vi "Save Setup.vi"(8 "error in (no error)":errorcluster, 11 "JSON in":refnum<class "JSON.lvclass">) -> (0 "error out":errorcluster, 3 "JSON out":refnum<class "JSON.lvclass">)   [LabVIEW 2018, in "JSON.lvclass"]
uses:
  JSON.lvclass
  JSON.lvclass/JSON.ctl
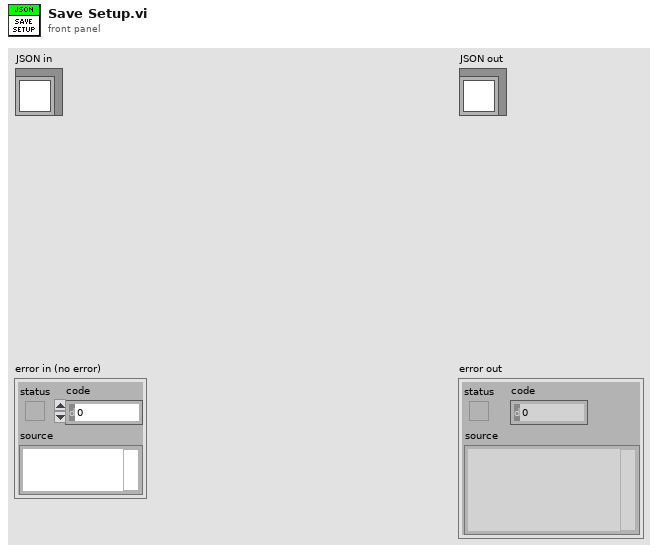
[diagram p1: front panel]
types:
  T1 = enum16{"open", "replace", "create", "open or create", "replace or create", "replace or create with confirmation"}
  T2 = cluster{"Exposure Time":dbl, "Readout Rate":u8, "Pre-amp gain":u8, "Initial Line":u16, "Final Line":u16, "Final Column":u16, "Initial Cloumn":u16, "Binning":u8, "EM Gain":u16, "EM Mode":u8, "Kinetic Series Length":u16}
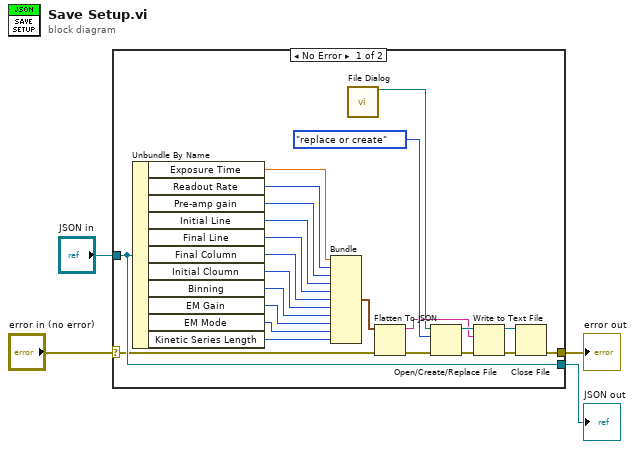
[diagram p0: block diagram]
diagram:
  n1 = case shown="No Error" "error in (no error)" {
    selector: "error in (no error)" -> [w14 w29]
    tunnel: [w7 w29] -> w3
    tunnel: [w27 w28] -> w1
    tunnel: "JSON in" -> [w27 w28]
    frame No Error {
      n2 = Unbundle By Name(w27) -> ("Exposure Time"=w26:dbl, "Readout Rate"=w24:u8, "Pre-amp gain"=w23:u8, "Initial Line"=w22:u16, "Final Line"=w21:u16, "Final Column"=w20:u16, "Initial Cloumn"=w19:u16, "Binning"=w18:u8, "EM Gain"=w17:u16, "EM Mode"=w16:u8, "Kinetic Series Length"=w15:u16)
      n3 = Bundle("Exposure Time"=w26, "Readout Rate"=w24, "Pre-amp gain"=w23, "Initial Line"=w22, "Final Line"=w21, "Final Column"=w20, "Initial Cloumn"=w19, "Binning"=w18, "EM Gain"=w17, "EM Mode"=w16, "Kinetic Series Length"=w15) -> (w25:T2)  [unwired: 1 in]
      n4 = call "File Dialog"() -> ("selected path"=w5:path)  [unwired: 12 in, 3 out]
      n5 = Flatten To JSON(anything=w25, error in (no error)=w14) -> (JSON string=w6:string, 11:w8:errorcluster)  [unwired: 1 in]
      n6 = Open/Create/Replace File(file path (use dialog)=w5, error in=w8, operation (0:open)=T1."replace or create") -> (refnum out=w11:refnum<file>, error out=w12:errorcluster)  [unwired: 3 in, 1 out]
      n7 = Write to Text File(file (use dialog)=w11, text=w6, error in=w12) -> (refnum out=w9:refnum<file>, error out=w10:errorcluster)  [unwired: 1 in, 1 out]
      n8 = Close File(refnum=w9, error in=w10) -> (error out=w7:errorcluster)  [unwired: 1 out]
    }
    frame Error {
    }
  }
  "error out" <- w3
  "JSON out" <- w1
